vi "BM0211-Image Editing.vi"(8 "error IN":errorcluster) -> (0 "error out":errorcluster)   [LabVIEW 2015]
uses:
  <vilib>/Utility/miscctls.llb/LVBoundsTypeDef.ctl
  <vilib>/Utility/miscctls.llb/LVPointTypeDef.ctl
panel:
  out "Assembly ST-1":picture
  out "filenames":string[](array[string])
  out "selected path":path
  out "Boolean":bool
  in  "Vertical position":sgl(slide) min=-2000 max=2000 scale=-1000.0..2000.0 scale format="%#.0f"
  in  "Horizontal position":sgl(slide) min=-2000 max=2000 scale=-1000.0..2000.0 scale format="%#.0f"
  in  "Zoom Factor":sgl(slide)=1.0 min=1 max=500 scale=0.0..500.0 scale format="%#.0f"
  out "2D Picture":picture
  in  "Stop Button":bool
  in  "Select Part":u16(ring) items=["P1.jpg", "P2.jpg", "P3.jpg", "P4.jpg", "P5.jpg", "P6.jpg", "P7.jpg", "P8.jpg", "P9.jpg", "P10.jpg", "P11.jpg", "P12.jpg"]
  in  "Save":bool
  in  "Select New":bool
  # "Image Editing"
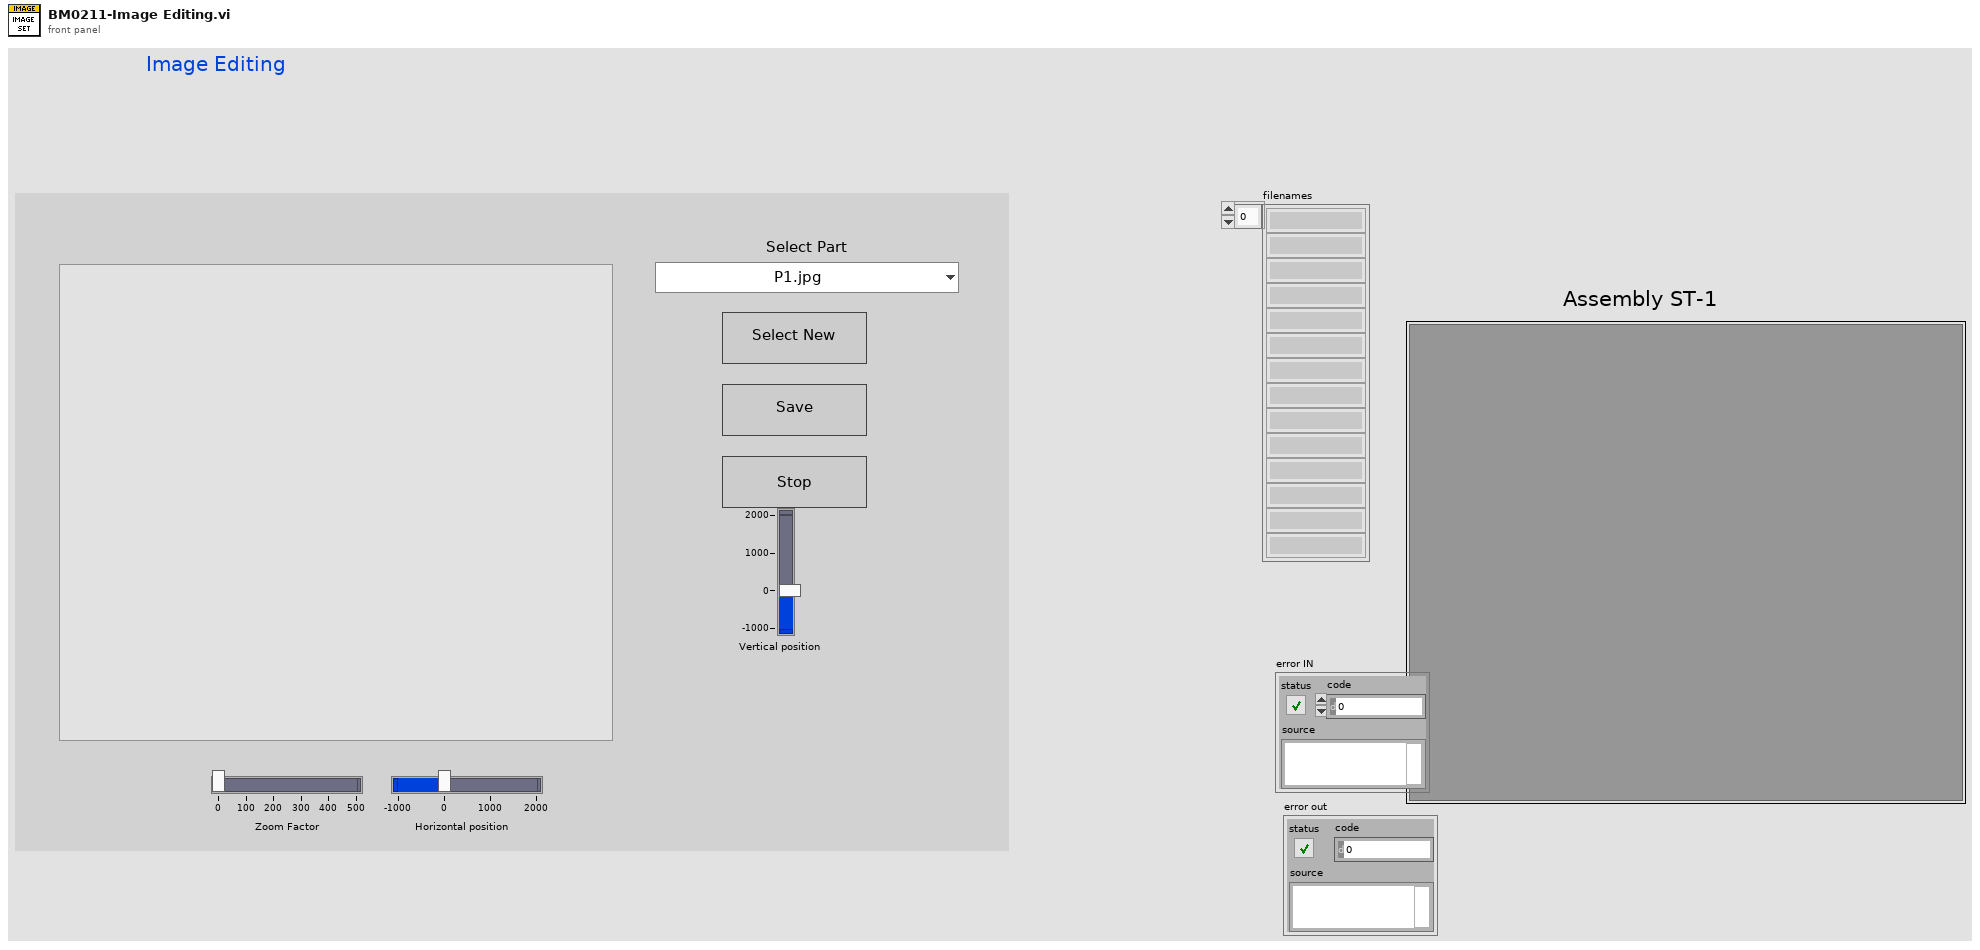
[diagram p1: front panel]
types:
  T1 = typedef "imagedata.ctl" = cluster{"image type":i32, "image depth":i32, "image":u8[], "mask":u8[], "colors":u32[], "Rectangle":cluster{"left":i16, "top":i16, "right":i16, "bottom":i16}}
  T2 = cluster{"Zoom Factor":sgl, "Horizontal position":sgl, "Vertical position":sgl}[]
  T3 = cluster{"Zoom Factor":sgl, "Horizontal position":sgl, "Vertical position":sgl}
  T4 = typedef "LVPointTypeDef.ctl" = cluster{"Horizontal":i16, "Vertical":i16}
  T5 = typedef "LVBoundsTypeDef.ctl" = cluster{"Width":u32, "Height":u32}
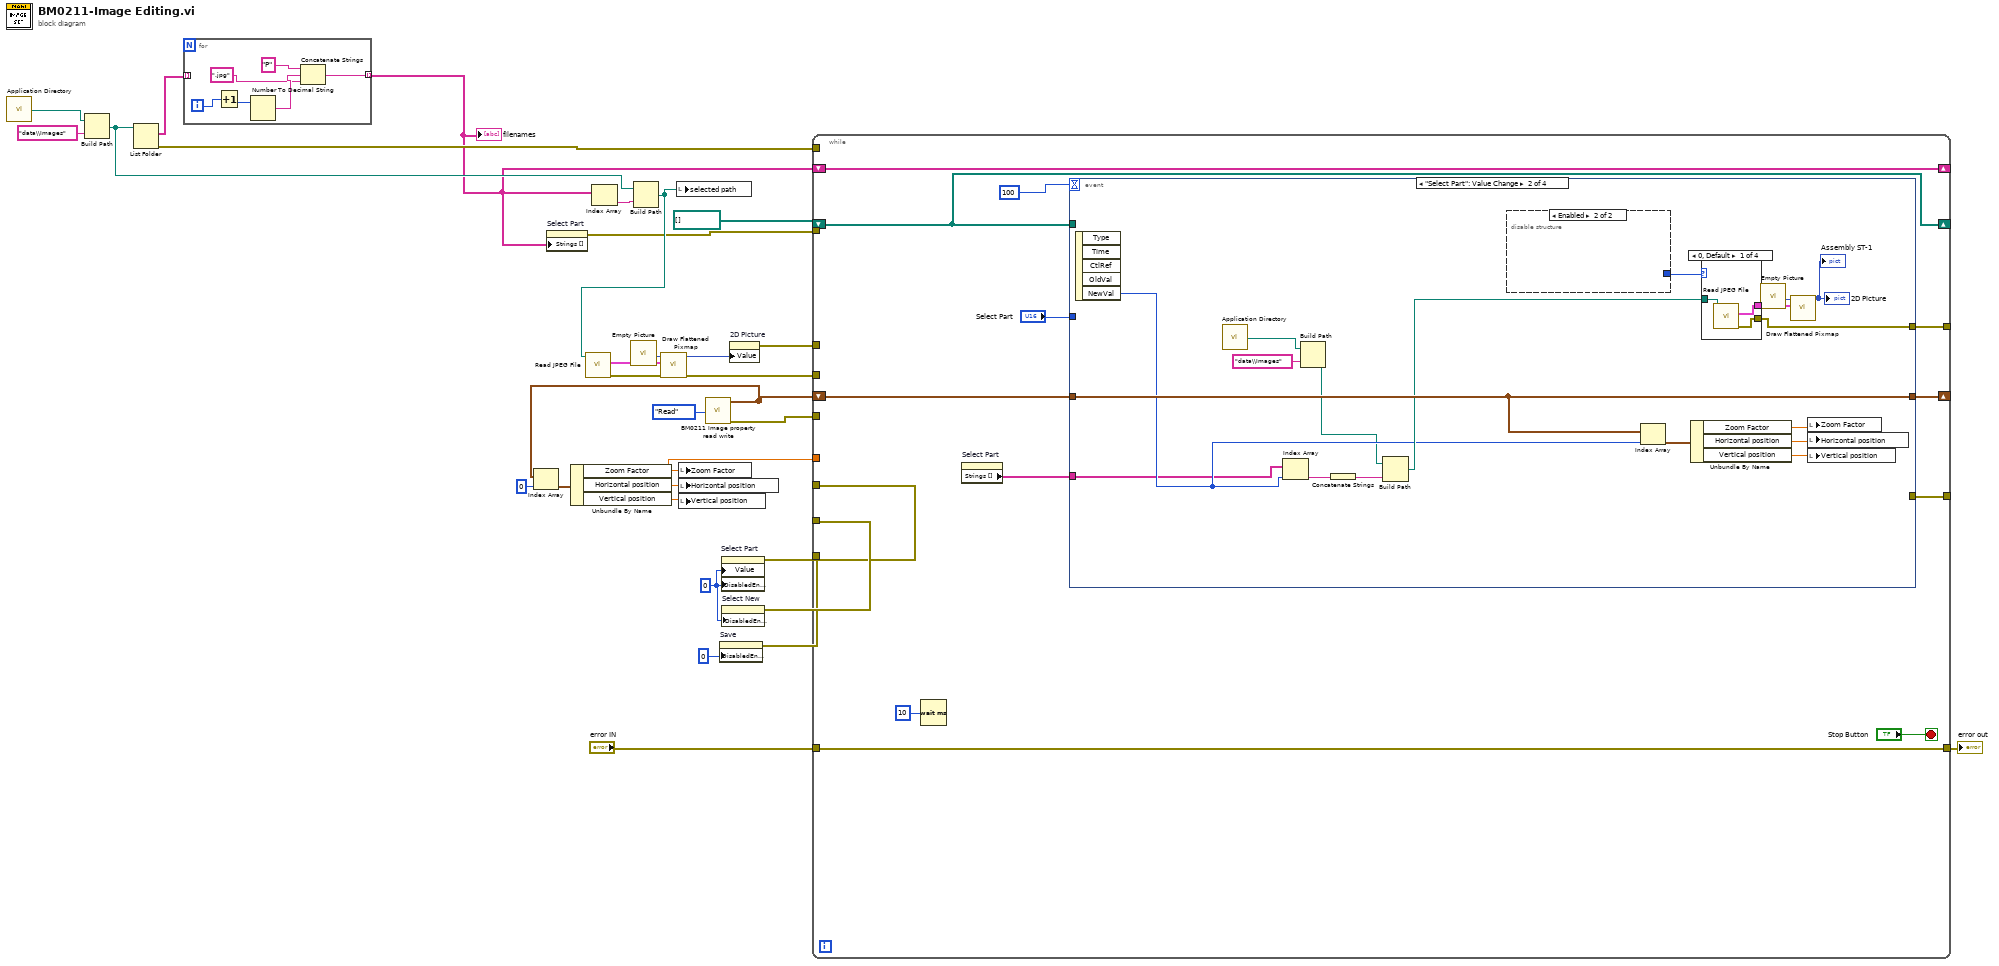
[diagram p0: block diagram]
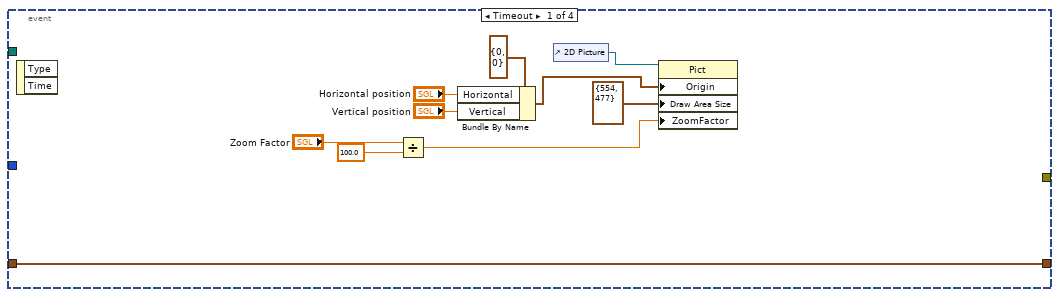
[diagram p2: hidden frame]
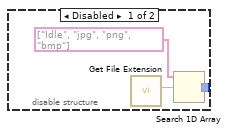
[diagram p3: hidden frame]
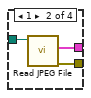
[diagram p4: hidden frame]
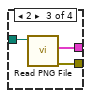
[diagram p5: hidden frame]
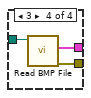
[diagram p6: hidden frame]
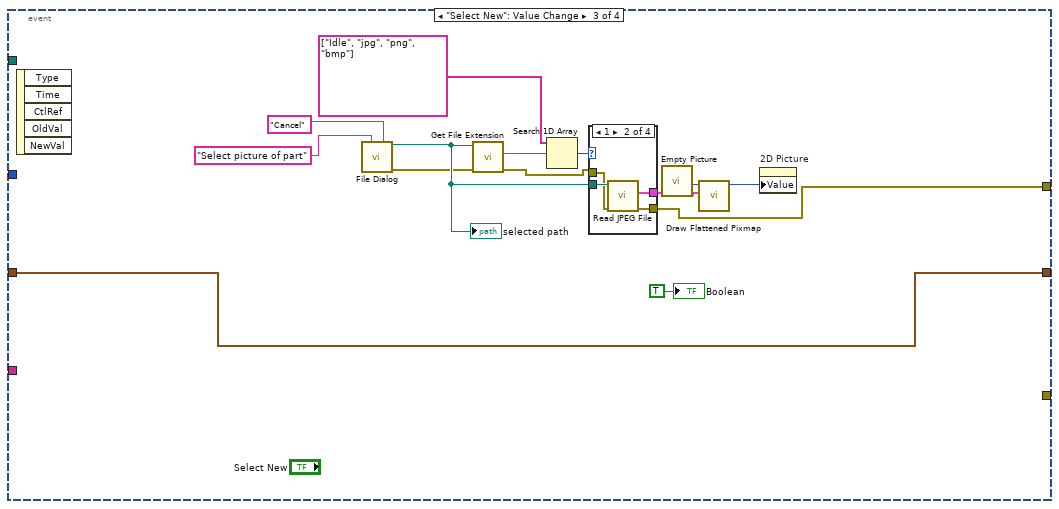
[diagram p7: hidden frame]
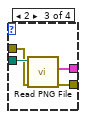
[diagram p9: hidden frame]
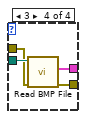
[diagram p10: hidden frame]
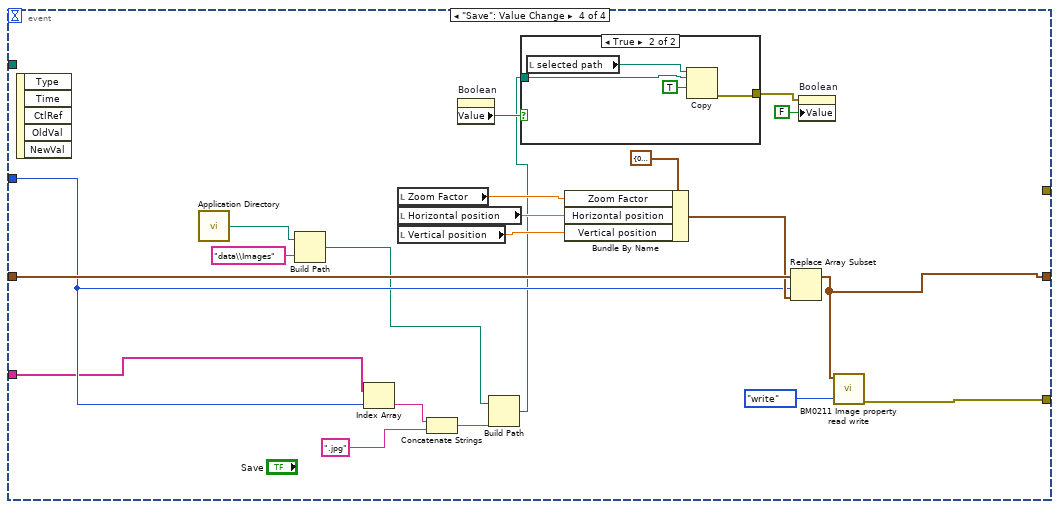
[diagram p11: hidden frame]
diagram:
  w14 = 0
  n1 = call <vilib>:"Application Directory.vi"() -> ("Application Directory"=w8:path)
  n2 = Build Path(base path=w8, name or relative path="data\\Images") -> (appended path=w6:path)
  n3 = List Folder(path=w6) -> (filenames=w2:string[], error out=w13:errorcluster)  [unwired: 3 in, 2 out]
  n4 = for {
    tunnel: w2 -> [_] mode=indexing
    tunnel: [w31] -> w1 mode=indexing
    i -> [w35]
    n5 = Increment(x=w35) -> (x+1=w36:i32)
    n6 = Number To Decimal String(number=w36) -> (decimal integer string=w34:string)  [unwired: 1 in]
    n7 = Concatenate Strings("P" ("string"), w34, ".jpg") -> (w31:string)
  }
  "filenames" <- w1
  n8 = property on="Select Part" class="Ring (strict)"("Strings []"=w1) -> (error out=w5:errorcluster)  [unwired: 2 in, 1 out]
  n9 = Index Array(array=w1) -> (element=w12:string)  [unwired: 1 in]
  n10 = call "Empty Picture"() -> ("empty picture"=w20:picture)
  n11 = Build Path(base path=w6, name or relative path=w12) -> (appended path=w9:path)
  n12 = call <vilib>:"Read JPEG File.vi"("path to JPEG file"=w9) -> ("error out"=w18:errorcluster, "image data"=w19:T1)  [unwired: 8 in, 1 out]
  n13 = call <vilib>:"Draw Flattened Pixmap.vi"("image data"=w19, "picture"=w20) -> ("new picture"=w17:picture)  [unwired: 7 in]
  n14 = local write "selected path"(w9) -> ()
  n15 = call "BM0211 Image property read write.vi"("Read write"=enum16{"write", "Read"}."Read") -> ("error out"=w10:errorcluster, "Out"=w23:T2)  [unwired: 9 in]
  n16 = Index Array(array=w23, index=0) -> (element=w24:T3)
  n17 = Unbundle By Name(w24) -> ("Zoom Factor"=w21:sgl, "Horizontal position"=w25:sgl, "Vertical position"=w26:sgl)
  n18 = local write "Zoom Factor"(w21) -> ()
  n19 = local write "Horizontal position"(w25) -> ()
  n20 = local write "Vertical position"(w26) -> ()
  n21 = property on="Save" class="Bool"("DisabledEnum"=0) -> (error out=w27:errorcluster)  [unwired: 2 in, 1 out]
  n22 = property on="Select Part" class="Ring (strict)"("Value"=w14, "DisabledEnum"=w14) -> (error out=w29:errorcluster)  [unwired: 2 in, 1 out]
  n23 = property on="Select New" class="Bool"("DisabledEnum"=w14) -> (error out=w30:errorcluster)  [unwired: 2 in, 1 out]
  n24 = property on="2D Picture" class="Pict"("Value"=w17) -> (error out=w16:errorcluster)  [unwired: 2 in, 1 out]
  n25 = while {
    shift-right: [w46] -> _
    shift-left: path[] [] ("Array") -> [w46]
    tunnel: [w45] -> _
    shift-right: [w42] -> _
    shift-left: w23 -> [w44]
    tunnel: w30 -> [_]
    tunnel: w29 -> [_]
    tunnel: w27 -> [_]
    tunnel: w21 -> [_]
    tunnel: w18 -> [_]
    tunnel: w16 -> [_]
    tunnel: w13 -> [_]
    shift-right: [w40] -> _
    shift-left: w1 -> [w40]
    tunnel: w10 -> [_]
    tunnel: [w39] -> _
    tunnel: w5 -> [_]
    tunnel: "error IN" -> [w37]
    tunnel: [w37] -> w3
    stop <- "Stop Button" stop-if-true
    n26 = Wait (ms)(milliseconds to wait=u32 10) -> ()  [unwired: 1 out]
    n27 = property on="Select Part" class="Ring (strict)"() -> ("Strings []"=w38:string[])  [unwired: 2 in, 2 out]
    n28 = event shown="[1] \"Select Part\": Value Change" {
      selector: _ -> [_ _ _ _]
      dyn-events: _ -> [_ _ _ _]
      timeout: 100 -> [_ _ _ _]
      tunnel: w46 -> [_ _ _ _]
      tunnel: [_ w75 w94 _] -> w45
      tunnel: w44 -> [w49 w72 w92 w132]
      tunnel: "Select Part" -> [_ _ _ w129]
      tunnel: [w49 w72 w92 w124] -> w42
      tunnel: [_ _ _ w127] -> w39
      tunnel: w38 -> [_ w60 _ w120]
      event Timeout {
        n29 = event-data() -> ()  [unwired: 1 in, 2 out]
        n30 = Divide(x="Zoom Factor", y=sgl 100.0 ("x")) -> (x/y=w55:sgl)
        n31 = Bundle By Name(cluster=T4 {"Horizontal"=0, "Vertical"=0} ("Origin"), "Horizontal"="Horizontal position", "Vertical"="Vertical position") -> (w51:T4)
        n32 = control-ref of="2D Picture"() -> (w56:refnum<vi>)
        n33 = property class="Pict"(reference=w56, "Origin"=w51, "Draw Area Size"=T5 {"Width"=554, "Height"=477}, "ZoomFactor"=w55) -> ()  [unwired: 1 in, 2 out]
      }
      event "Select Part": Value Change {
        n34 = event-data() -> ("NewVal"=w64:u16)  [unwired: 1 in, 4 out]
        n35 = call <vilib>:"Application Directory.vi"() -> ("Application Directory"=w63:path)
        n36 = Index Array(array=w60, index=w64) -> (element=w67:string)
        n37 = Build Path(base path=w63, name or relative path="data\\Images") -> (appended path=w61:path)
        n38 = Concatenate Strings(w67) -> (w65:string)
        n39 = Build Path(base path=w61, name or relative path=w65) -> (appended path=w66:path)
        n40 = disable-structure shown="Enabled" {
          disable-tunnel: [w77 _] -> w74
          frame Disabled {
            n41 = call <vilib>:"Get File Extension.vi"() -> ("lowercase file extension"=w78:string)  [unwired: 7 in, 4 out]
            n42 = Search 1D Array(1D array=string[] ["Idle", "jpg", "png", "bmp"] ("Strings []"), element=w78) -> (index of element=w77:i32)  [unwired: 1 in]
          }
          frame Enabled {
          }
        }
        n43 = Index Array(array=w72, index=w64) -> (element=w71:T3)
        n44 = Unbundle By Name(w71) -> ("Zoom Factor"=w70:sgl, "Horizontal position"=w69:sgl, "Vertical position"=w68:sgl)
        n45 = case shown="0, Default" w74 {
          tunnel: [w81 w85 w87 w90] -> w73
          tunnel: [w80 w84 w86 w91] -> w75
          tunnel: w66 -> [w82 w83 w88 w89]
          frame 0, Default {
            n46 = call <vilib>:"Read JPEG File.vi"("path to JPEG file"=w82) -> ("error out"=w80:errorcluster, "image data"=w81:T1)  [unwired: 8 in, 1 out]
          }
          frame 1 {
            n47 = call <vilib>:"Read JPEG File.vi"("path to JPEG file"=w83) -> ("error out"=w84:errorcluster, "image data"=w85:T1)  [unwired: 8 in, 1 out]
          }
          frame 2 {
            n48 = call <vilib>:"Read PNG File.vi"("path to PNG file"=w88) -> ("error out"=w86:errorcluster, "image data"=w87:T1)  [unwired: 8 in, 1 out]
          }
          frame 3 {
            n49 = call <vilib>:"Read BMP File.vi"("path to BMP file"=w89) -> ("error out"=w91:errorcluster, "image data"=w90:T1)  [unwired: 8 in, 1 out]
          }
        }
        n50 = call "Empty Picture"() -> ("empty picture"=w76:picture)
        n51 = call <vilib>:"Draw Flattened Pixmap.vi"("image data"=w73, "picture"=w76) -> ("new picture"=→"2D Picture" →"Assembly ST-1":picture)  [unwired: 7 in]
        n52 = local write "Zoom Factor"(w70) -> ()
        n53 = local write "Horizontal position"(w69) -> ()
        n54 = local write "Vertical position"(w68) -> ()
      }
      event "Select New": Value Change {
        n55 = event-data() -> ()  [unwired: 1 in, 5 out]
        n56 = call "File Dialog"("prompt"="Select picture of part", "button label"="Cancel") -> ("selected path"=w97:path, "error out"=w96:errorcluster)  [unwired: 10 in, 2 out]
        "selected path" <- w97
        n57 = call <vilib>:"Get File Extension.vi"("error in (no error)"=w96, "file"=w97) -> ("error out"=w101:errorcluster, "lowercase file extension"=w103:string)  [unwired: 5 in, 3 out]
        n58 = Search 1D Array(1D array=string[] ["Idle", "jpg", "png", "bmp"] ("Strings []"), element=w103) -> (index of element=w102:i32)  [unwired: 1 in]
        n59 = case shown="1" w102 {
          tunnel: [_ w110 w114 w117] -> w95
          tunnel: [w106 w109 w113 w118] -> w94
          tunnel: w101 -> [w106 w107 w111 w115]
          tunnel: w97 -> [_ w108 w112 w116]
          frame 0, Default {
          }
          frame 1 {
            n60 = call <vilib>:"Read JPEG File.vi"("error in (no error)"=w107, "path to JPEG file"=w108) -> ("error out"=w109:errorcluster, "image data"=w110:T1)  [unwired: 7 in, 1 out]
          }
          frame 2 {
            n61 = call <vilib>:"Read PNG File.vi"("error in (no error)"=w111, "path to PNG file"=w112) -> ("error out"=w113:errorcluster, "image data"=w114:T1)  [unwired: 7 in, 1 out]
          }
          frame 3 {
            n62 = call <vilib>:"Read BMP File.vi"("error in (no error)"=w115, "path to BMP file"=w116) -> ("error out"=w118:errorcluster, "image data"=w117:T1)  [unwired: 7 in, 1 out]
          }
        }
        n63 = call "Empty Picture"() -> ("empty picture"=w105:picture)
        n64 = call <vilib>:"Draw Flattened Pixmap.vi"("image data"=w95, "picture"=w105) -> ("new picture"=w100:picture)  [unwired: 7 in]
        n65 = property on="2D Picture" class="Pict"("Value"=w100) -> ()  [unwired: 2 in, 2 out]
        "Boolean" <- TRUE
      }
      event "Save": Value Change {
        n66 = event-data() -> ()  [unwired: 1 in, 5 out]
        n67 = call <vilib>:"Application Directory.vi"() -> ("Application Directory"=w123:path)
        n68 = Build Path(base path=w123, name or relative path="data\\Images") -> (appended path=w121:path)
        n69 = Index Array(array=w120, index=w129) -> (element=w119:string)
        n70 = local read "Zoom Factor"() -> (w136:sgl)
        n71 = local read "Horizontal position"() -> (w135:sgl)
        n72 = local read "Vertical position"() -> (w134:sgl)
        n73 = Concatenate Strings(w119, ".jpg" ("string")) -> (w126:string)
        n74 = property on="Boolean" class="Bool (strict)"() -> ("Value"=w139:bool)  [unwired: 2 in, 2 out]
        n75 = Build Path(base path=w121, name or relative path=w126) -> (appended path=w128:path)
        n76 = case shown="True" w139 {
          tunnel: w128 -> [_ w140]
          tunnel: [_ w143] -> w137
          frame False {
          }
          frame True {
            n77 = local read "selected path"() -> (w142:path)
            n78 = Copy(9:TRUE ("overwrite (F)"), 10:w140, 11:w142) -> (0:w143:errorcluster)  [unwired: 2 in, 2 out]
          }
        }
        n79 = Bundle By Name(cluster=T3 {"Zoom Factor"=0.0, "Horizontal position"=0.0, "Vertical position"=0.0} ("element"), "Zoom Factor"=w136, "Horizontal position"=w135, "Vertical position"=w134) -> (w131:T3)
        n80 = Replace Array Subset(array=w132, new element=w131, index=w129) -> (w124:T2)
        n81 = property on="Boolean" class="Bool (strict)"(error in=w137, "Value"=FALSE ("Boolean")) -> ()  [unwired: 1 in, 2 out]
        n82 = call "BM0211 Image property read write.vi"("Read write"=enum16{"write", "Read"}."write", "IN"=w124) -> ("error out"=w127:errorcluster)  [unwired: 8 in, 1 out]
      }
    }
  }
  "error out" <- w3
